vi "LAInitSession.vi"(8 "Error In":errorcluster, 10 "AgentId":string, 11 "LiteAgent In":T1) -> (0 "Error Out":errorcluster, 2 "SessionId":string, 3 "LiteAgent Out":T1)   [LabVIEW 2017, in "LiteAgentSDK.lvlib"]
uses:
  LiteAgentSDK.lvlib
  C:/Users/Jan/Projects/LiteAgentSDK-LabVIEW/Source/Bin/LiteAgentSDK.LabVIEW.dll
  Bin/LiteAgentSDK.LabVIEW.dll
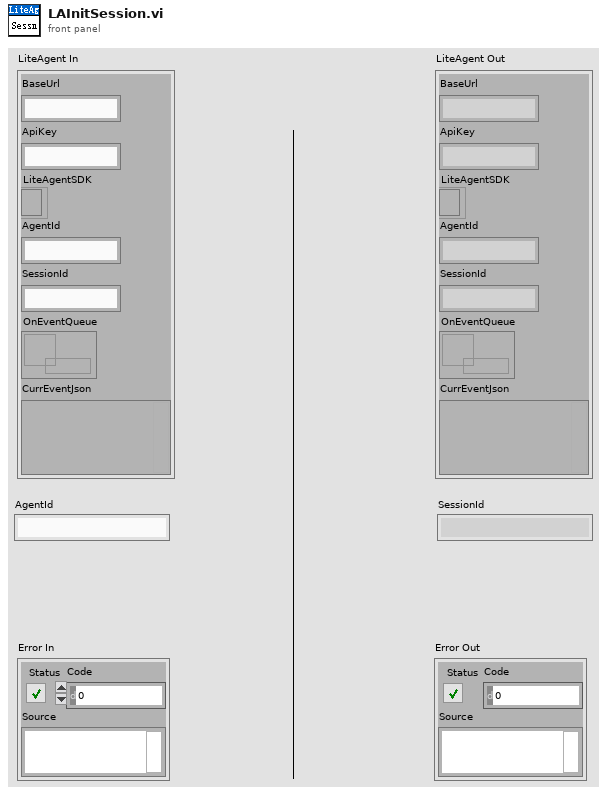
[diagram p1: front panel]
types:
  T1 = cluster{"BaseUrl":string, "ApiKey":string, "LiteAgentSDK":refnum<k24>, "AgentId":string, "SessionId":string, "OnEventQueue":refnum<queue>, "CurrEventJson":variant}
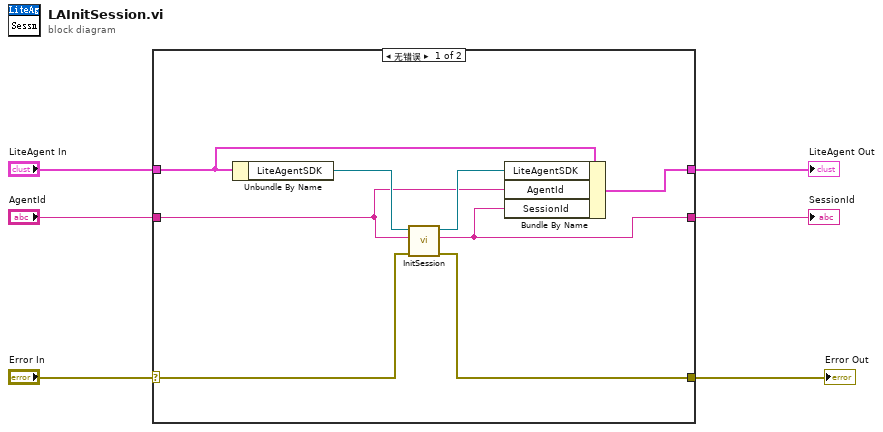
[diagram p0: block diagram]
diagram:
  n1 = case shown="无错误" "Error In" {
    selector: "Error In" -> [w14 w16]
    tunnel: [w13 w16] -> w5
    tunnel: "AgentId" -> [w10 _]
    tunnel: "LiteAgent In" -> [w8 w15]
    tunnel: [w9 w15] -> w2
    tunnel: [w7 _] -> w1
    frame No Error {
      n2 = Unbundle By Name(w8) -> ("LiteAgentSDK"=w12:refnum<k24>)
      n3 = call "InitSession.vi"("Error Input"=w14, "AgentId"=w10, "LiteAgentSDK Input"=w12) -> ("Error Output"=w13:errorcluster, "sessionId"=w7:string, "LiteAgentSDK Output"=w11:refnum<k24>)  [unwired: 6 in]
      n4 = Bundle By Name(cluster=w8, "LiteAgentSDK"=w11, "AgentId"=w10, "SessionId"=w7) -> (w9:T1)
    }
    frame Error {
    }
  }
  "Error Out" <- w5
  "LiteAgent Out" <- w2
  "SessionId" <- w1
